vi "Pre Launch Init.vi"(11 "VolatusCore in":refnum<class "VolatusCore.lvclass">) -> (0 "error out":errorcluster, 3 "VolatusCore out":refnum<class "VolatusCore.lvclass">)   [LabVIEW 2020, in "Volatus.lvlib" / "VolatusCore.lvclass"]
doc: "(<B>Filename</B>: Actor Framework.lvlib:Actor.lvclass:Pre Launch Init.vi)\n\nDefines behavior that occurs after the Launch Nested Actor method is invoked but before the actor's Actor Core method begins running.\n\nBy default, this method does nothing. A descendant class may override it to define behavior."
uses:
  VolatusCore.lvclass
  C:/Program Files (x86)/National Instruments/LabVIEW 2020/vi.lib/ActorFramework/Actor/Actor.lvclass
  Startup Notification.ctl
  App/App.lvclass
  Core APIs.ctl
  VolatusAPI/VolatusAPI.lvclass
  C:/dev/lv20CE/relink/lv-volatus/Volatus/API/API.lvclass
  <vilib>/ActorFramework/Actor/Actor.lvclass/Actor.ctl
  <vilib>/ActorFramework/Message Enqueuer/Message Enqueuer.lvclass/Message Enqueuer.ctl
  VolatusCore.lvclass/VolatusCore.ctl
  <vilib>/ActorFramework/Message Enqueuer/Init from Existing Queue.vi
  <vilib>/ActorFramework/Message Enqueuer/Enqueue.vi
  VolatusCore Messages/Startup Msg/Startup Msg.lvclass
  C:/Program Files (x86)/National Instruments/LabVIEW 2020/vi.lib/ActorFramework/Message/Message.lvclass
  <vilib>/ActorFramework/Message Priority Queue/Priority Enqueue.vi
  <vilib>/ActorFramework/Message Enqueuer/Message Enqueuer.lvclass
  <vilib>/ActorFramework/Actor/Actor.lvclass
  Volatus.lvlib
  C:/dev/lv20CE/relink/lv-volatus/Volatus/VolatusCore/VolatusCore.lvclass
  C:/dev/lv20CE/relink/lv-volatus/Volatus/TaskStateHandler/TaskStateHandler.lvclass
  C:/dev/lv20CE/relink/lv-volatus/Volatus/VectoMessageHandler/VectoMessageHandler.lvclass
  C:/dev/lv20CE/relink/lv-volatus/Volatus/VolatusAPI/VolatusAPI.lvclass
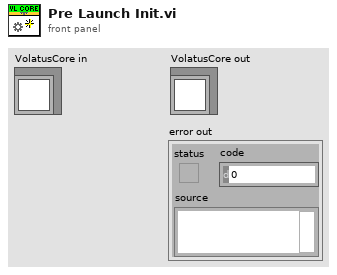
[diagram p1: front panel]
types:
  T1 = typedef "Volatus.lvlib/VolatusCore.lvclass/Startup Notification.ctl" = cluster{"Start":bool, "App":refnum<class "App.lvclass">, "Core APIs":T2}
  T2 = typedef "Volatus.lvlib/Core APIs.ctl" = cluster{"Volatus":refnum<class "VolatusAPI.lvclass">}
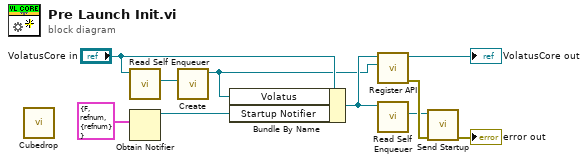
[diagram p0: block diagram]
diagram:
  n1 = call "Cubedrop.vi"() -> ()  [unwired: 12 in]
  n2 = call <vilib>:"Read Self Enqueuer.vi"("Actor"="VolatusCore in") -> ("Self Enqueuer"=w9:refnum<class "Message Enqueuer.lvclass">)  [unwired: 10 in]
  n3 = Obtain Notifier(notification data type=T1 {"Start"=FALSE, "App"=refnum, "Core APIs"={"Volatus"=refnum}} ("Startup Notification")) -> (notifier out=w7:refnum<notifier>)  [unwired: 3 in, 2 out]
  n4 = call "Create.vi"("EnQr"=w9) -> ("VolatusAPI out"=w1:refnum<class "VolatusAPI.lvclass">)  [unwired: 9 in, 1 out]
  n5 = Bundle By Name(cluster="VolatusCore in", "Volatus"=w1, "Startup Notifier"=w7) -> (w2:refnum<class "VolatusCore.lvclass">)
  n6 = call "Register API.vi"("API"=w1, "VolatusCore in"=w2) -> ("error out"=w10:errorcluster, "VolatusCore out"=→"VolatusCore out":refnum<class "VolatusCore.lvclass">)  [unwired: 8 in]
  n7 = call <vilib>:"Read Self Enqueuer.vi"("Actor"=w2) -> ("Self Enqueuer"=w6:refnum<class "Message Enqueuer.lvclass">)  [unwired: 10 in]
  n8 = call "Send Startup.vi"("error in (no error)"=w10, "Message Enqueuer"=w6) -> ("error out"=→"error out":errorcluster)  [unwired: 8 in, 1 out]
